vi "Add Terminating Bytes.vi"(11 "Size of Data":u64) -> (1 "Extra bytes":u64, 2 "Number of Chunks":u64, 3 "Array":u8[](array[numeric]))   [LabVIEW 2018, in "SHA256.lvlib"]
uses:
  SHA256.lvlib
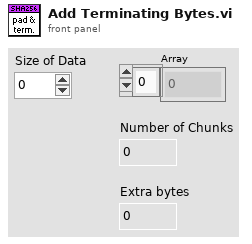
[diagram p1: front panel]
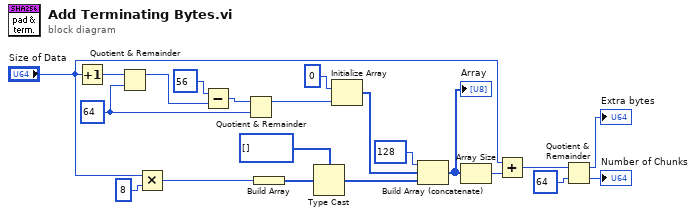
[diagram p0: block diagram]
diagram:
  w12 = 64 ("y")
  n1 = Increment(x="Size of Data") -> (x+1=w2:u64)
  n2 = Quotient & Remainder(x=w2, y=w12) -> (x-y*floor(x/y)=w3:u64)  [unwired: 1 out]
  n3 = Multiply(x="Size of Data", y=u64 8) -> (x*y=w14:u64)
  n4 = Subtract(x=56, y=w3) -> (x-y=w11:u64)
  n5 = Quotient & Remainder(x=w11, y=w12) -> (x-y*floor(x/y)=w17:u64)  [unwired: 1 out]
  n6 = Build Array(w14) -> (w15:u64[])
  n7 = Type Cast(type=u8[] [] ("unsigned byte array"), x=w15) -> (*(type *) &x=w16:u8[])
  n8 = Initialize Array(u8 0, w17) -> (w6:u8[])
  n9 = Build Array (concatenate)(u8 128, w6, w16) -> (w19:u8[])
  "Array" <- w19
  n10 = Array Size(array=w19) -> (size(s)=w8:i32)
  n11 = Add(x="Size of Data", y=w8) -> (x+y=w20:u64)
  n12 = Quotient & Remainder(x=w20, y=u64 64) -> (x-y*floor(x/y)=→"Extra bytes":u64, floor(x/y)=→"Number of Chunks":u64)
